vi "5T_Split_Cluster.vi"(0 "5 T Cluster":T2 {"Rate (T/min)" format="%6_5f"; "Leads (T)" format="%6_5f"}) -> (1 "5 T Status":T1 {"Leads (T)" format="%#_6f"}, 2 "5T Control":T3 {"Rate (T/min)" format="%6_5f"})   [LabVIEW 2019]
uses:
  Mischer/5T_Control.ctl
  Mischer/5T-Cluster.ctl
  Mischer/5T_Status.ctl
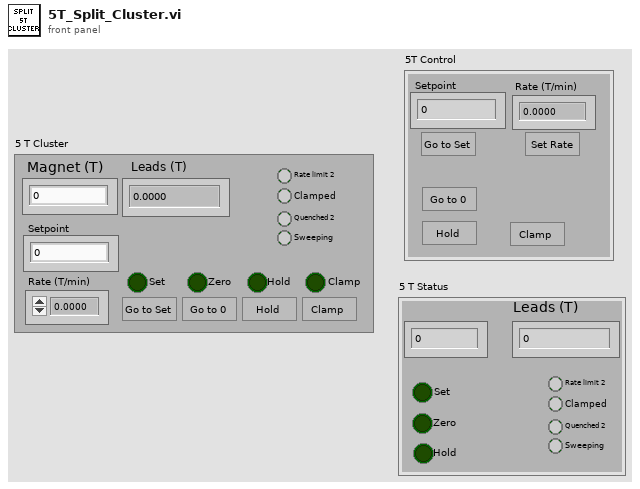
[diagram p1: front panel]
types:
  T1 = typedef "5T_Status.ctl" = cluster{"Magnet (T)":dbl, "Leads (T)":dbl, "Clamped ":bool, "Quenched 2":bool, "Rate limit 2":bool, "Sweeping":bool, "Set":bool, "Zero":bool, "Hold":bool}
  T2 = typedef "5T-Cluster.ctl" = cluster{"Go to set":bool, "Go to Zero":bool, "Clamp":bool, "Go to Hold":bool, "Clamped ":bool, "Quenched 2":bool, "Rate limit 2":bool, "Magnet (T)":dbl, "Leads (T)":dbl, "Rate (T/min)":dbl, "Sweeping":bool, "Setpoint":dbl, "Set":bool, "Zero":bool, "Hold":bool, "Clamp":bool}
  T3 = typedef "5T_Control.ctl" = cluster{"Rate (T/min)":dbl, "Setpoint":dbl, "Go to set":bool, "Go to Zero":bool, "Clamp":bool, "Go to Hold":bool, "Set Rate":bool}
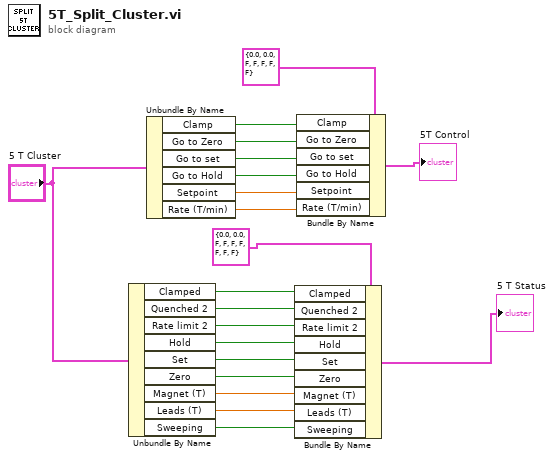
[diagram p0: block diagram]
diagram:
  n1 = Unbundle By Name("5 T Cluster") -> ("Clamped"=w9:bool, "Quenched 2"=w8:bool, "Rate limit 2"=w7:bool, "Hold"=w6:bool, "Set"=w5:bool, "Zero"=w4:bool, "Magnet (T)"=w3:dbl, "Leads (T)"=w2:dbl, "Sweeping"=w1:bool)
  n2 = Unbundle By Name("5 T Cluster") -> ("Clamp"=w18:bool, "Go to Zero"=w17:bool, "Go to set"=w16:bool, "Go to Hold"=w15:bool, "Setpoint"=w14:dbl, "Rate (T/min)"=w13:dbl)
  n3 = Bundle By Name(cluster=T1 {"Magnet (T)"=0.0, "Leads (T)"=0.0, "Clamped "=FALSE, "Quenched 2"=FALSE, "Rate limit 2"=FALSE, "Sweeping"=FALSE, "Set"=FALSE, "Zero"=FALSE, "Hold"=FALSE} ("5 T Status 2"), "Clamped"=w9, "Quenched 2"=w8, "Rate limit 2"=w7, "Hold"=w6, "Set"=w5, "Zero"=w4, "Magnet (T)"=w3, "Leads (T)"=w2, "Sweeping"=w1) -> (→"5 T Status":T1)
  n4 = Bundle By Name(cluster=T3 {"Rate (T/min)"=0.0, "Setpoint"=0.0, "Go to set"=FALSE, "Go to Zero"=FALSE, "Clamp"=FALSE, "Go to Hold"=FALSE, "Set Rate"=FALSE} ("5T Control"), "Clamp"=w18, "Go to Zero"=w17, "Go to set"=w16, "Go to Hold"=w15, "Setpoint"=w14, "Rate (T/min)"=w13) -> (→"5T Control":T3)
